vi "GxSingleCam.vi"() -> ()   [LabVIEW 2013]
uses:
  C:/Program Files/Daheng Imaging/GalaxySDK/Samples/LabVIEW SDK/x64/GxLVLib/dll/GxIAPINET.dll
  GxLVLib/dll/GxIAPINET.dll
  <vilib>/vision/Image Controls.llb/IMAQ Image.ctl
  GxLVLib/GxLVlib.lvlib
panel:
  out "IsExit":bool
  in  "Image Path":path
  in  "ImageSaving":bool
  in  "Image Src":T1
  out "Image":T1(plugin-control)
  out "Acquisition Callback":refnum<k27>
  out "IsColor":bool
  out "Acquisition Status":bool
  out "Open Status":bool
  in  "IGxFactory":refnum<k24>
  in  "Exit":bool
  in  "IGxStream":refnum<k24>
  in  "IGxDevice":refnum<k24>
  out "error out":errorcluster
  in  "TriggerSoftware":bool
  in  "BalanceWhiteAuto":string(combo)
  in  "Gain":dbl format="%#_6f"
  in  "ExposureTime":dbl
  in  "TriggerSource":string(combo)
  in  "TriggerMode":string(combo)
  in  "Acquisition Stop":bool
  in  "Acquisition Start":bool
  in  "Close Device":bool
  in  "Open Device":bool
  # "TriggerMode"
  # "TriggerSource"
  # "TriggerSoftware"
  # "ExposureTime(us)"
  # "Gain(dB)"
  # "BalanceWhiteAuto"
  # "ImageSaving"
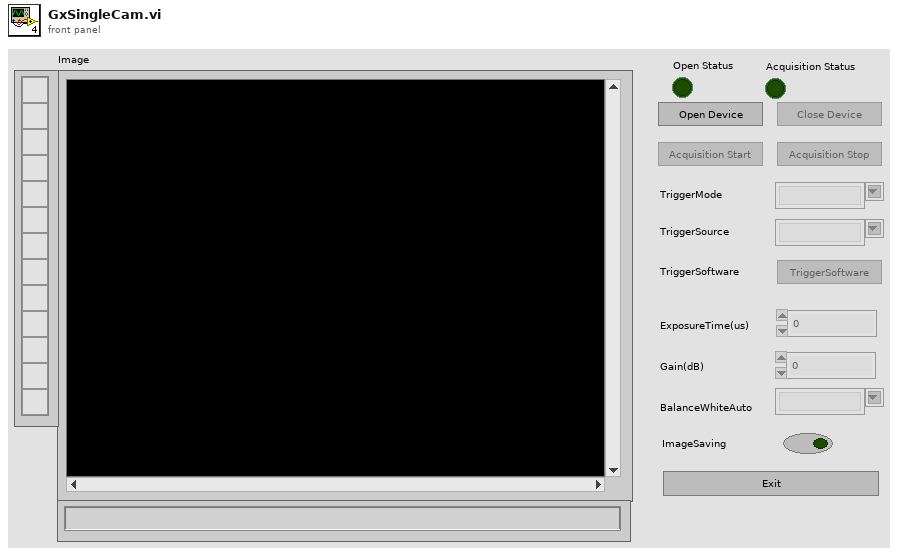
[diagram p1: front panel]
types:
  T1 = typedef "IMAQ Image.ctl" = refnum<image>
  T2 = typedef "Semaphore RefNum" = refnum<k1>
  T3 = enum8{"Enabled", "Disabled", "Disabled and Grayed Out"}
  T4 = typedef "Image Type" = u32
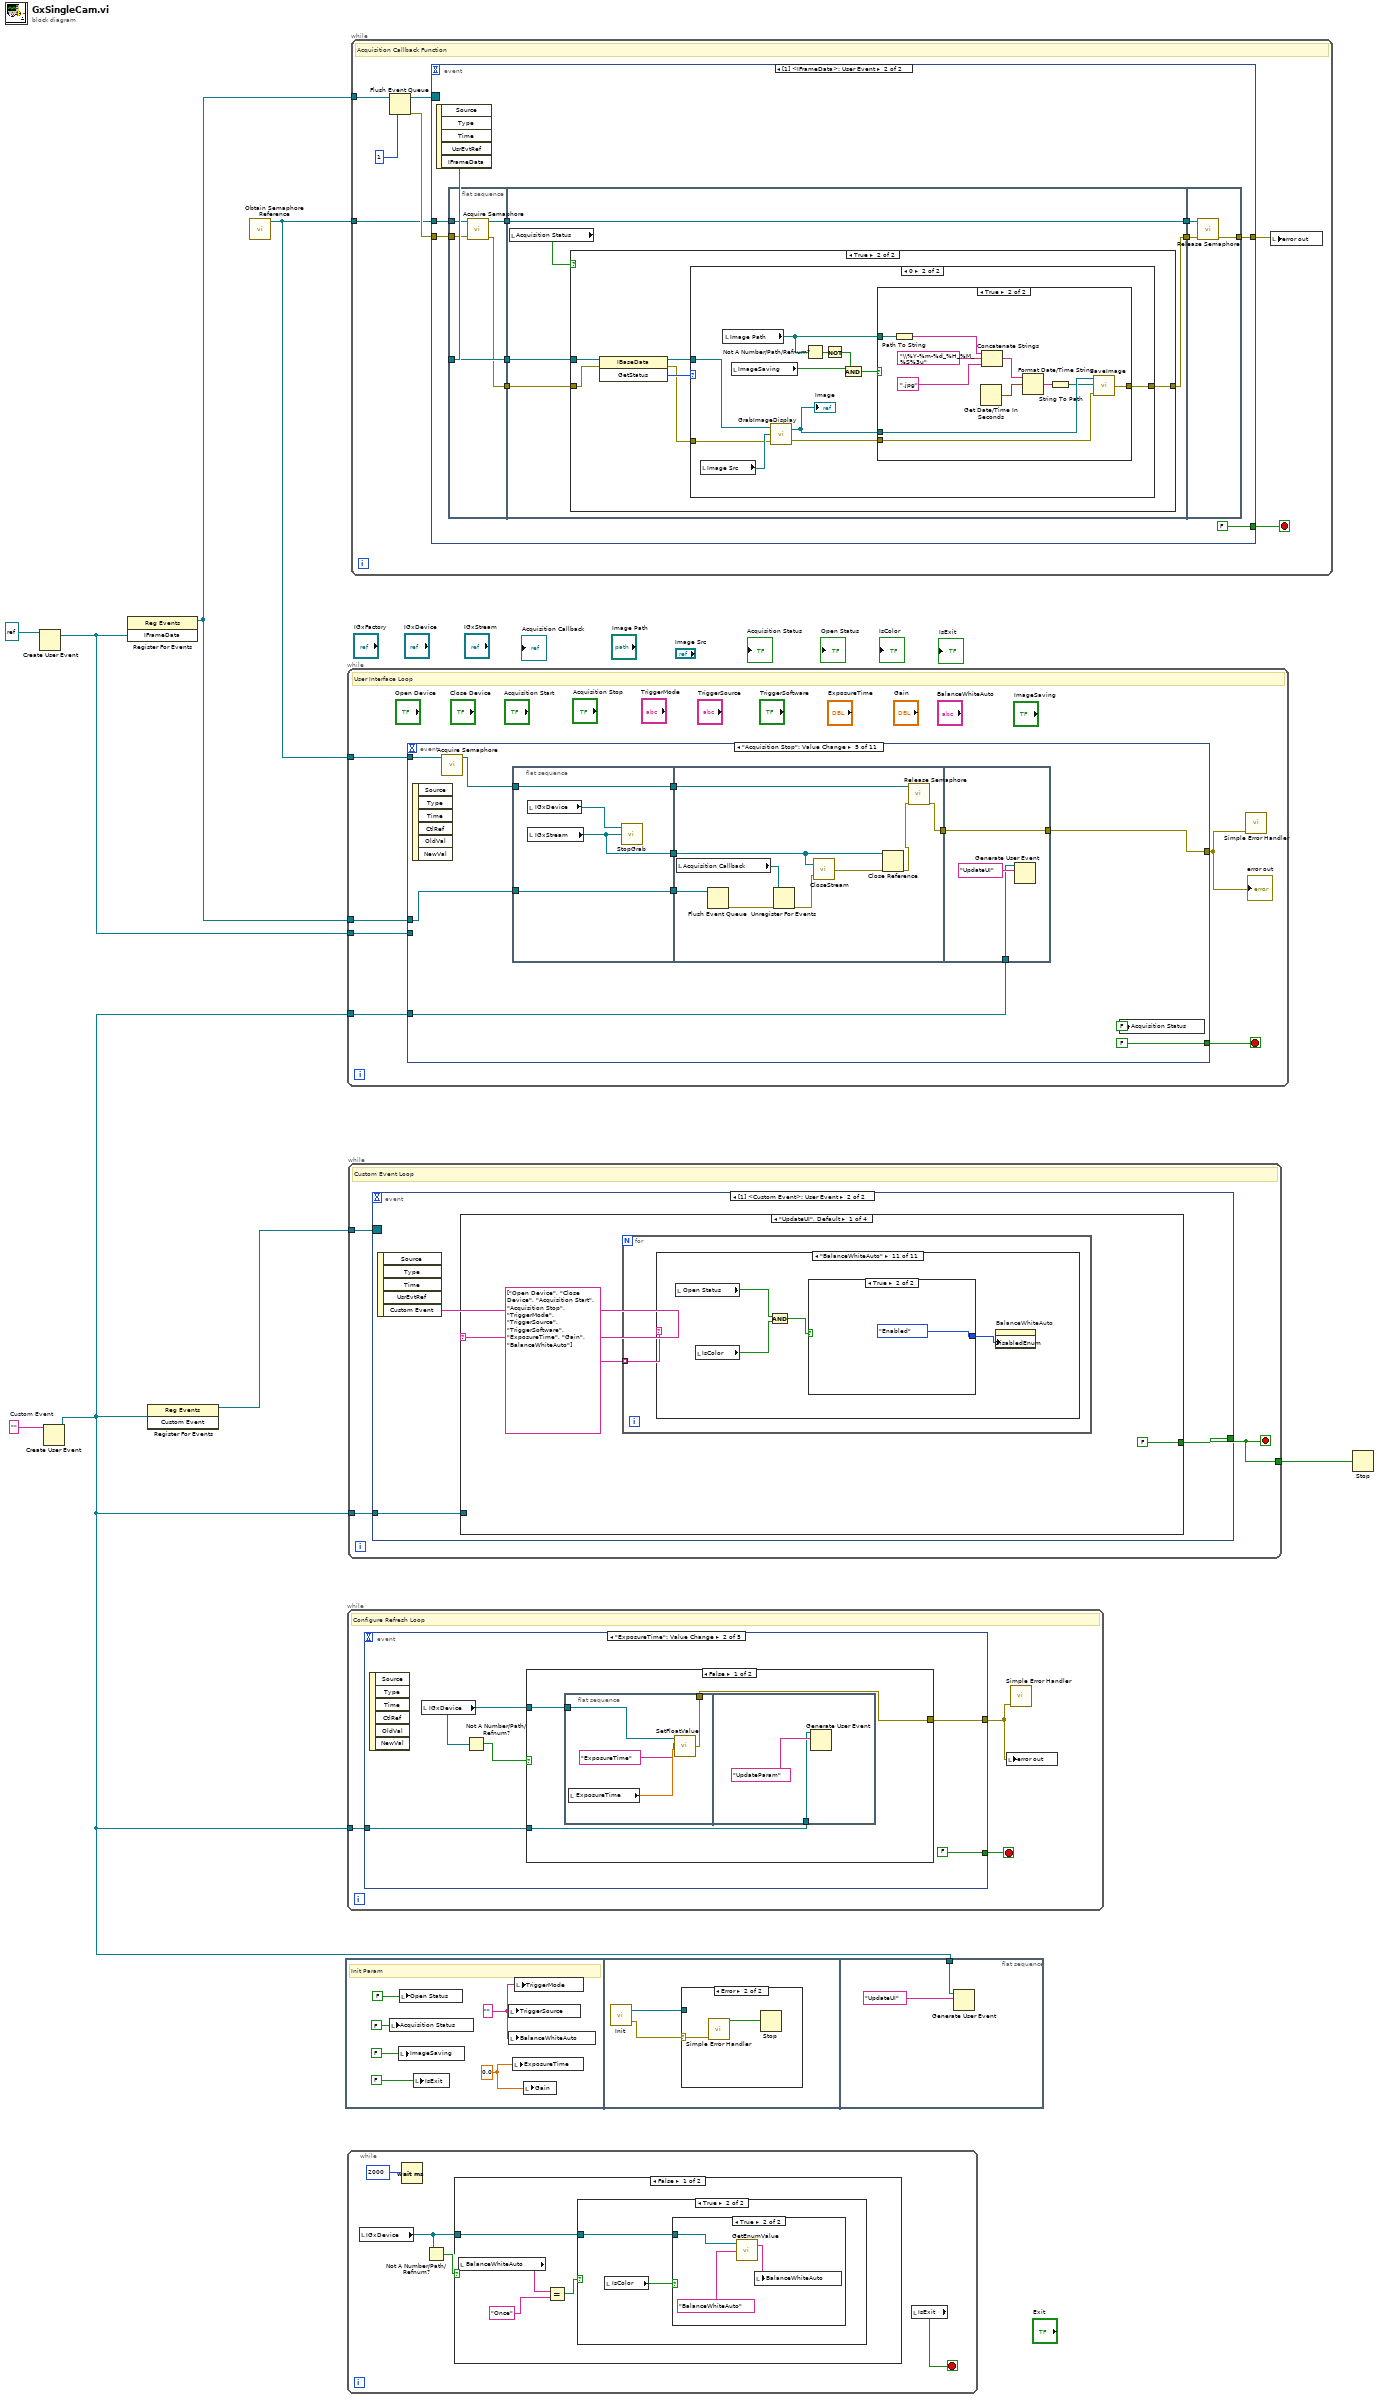
[diagram p0: block diagram]
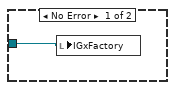
[diagram p5: hidden frame]
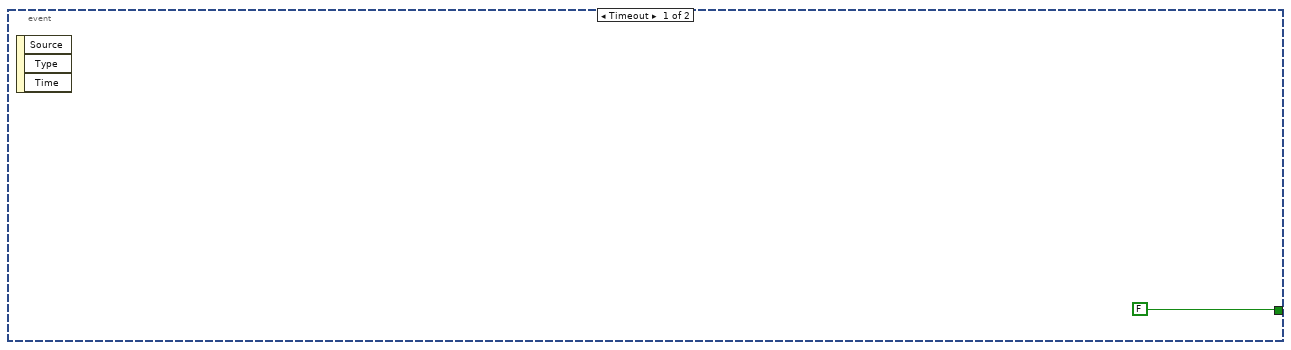
[diagram p6: hidden frame]
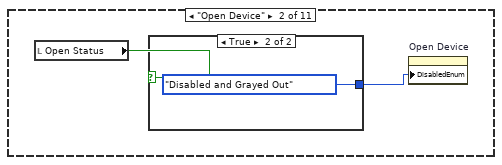
[diagram p8: hidden frame]
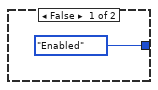
[diagram p9: hidden frame]
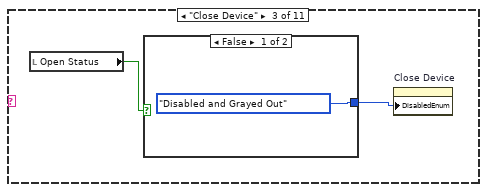
[diagram p10: hidden frame]
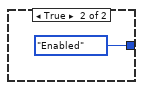
[diagram p11: hidden frame]
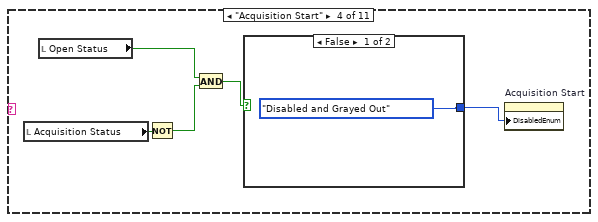
[diagram p12: hidden frame]
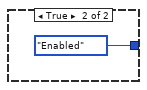
[diagram p13: hidden frame]
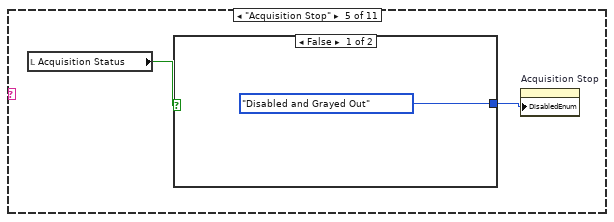
[diagram p14: hidden frame]
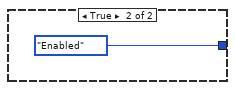
[diagram p15: hidden frame]
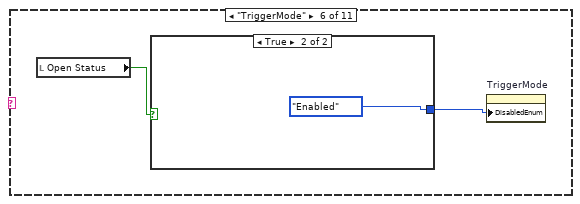
[diagram p16: hidden frame]
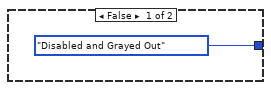
[diagram p17: hidden frame]
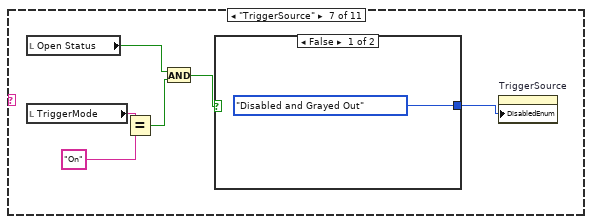
[diagram p18: hidden frame]
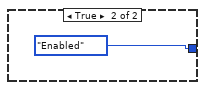
[diagram p19: hidden frame]
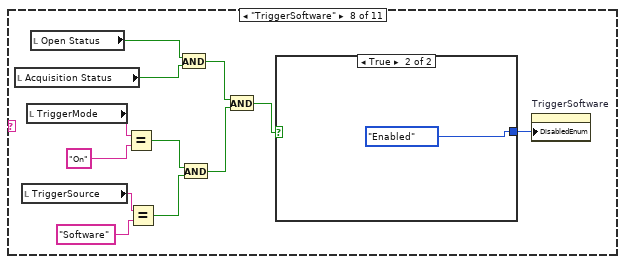
[diagram p20: hidden frame]
diagram:
  w6 = ""  # Custom Event
  n1 = Create User Event(user event datatype=refnum<k24> refnum ("IFrameData")) -> (user event=w8:refnum<user-event>)  [unwired: 1 in, 1 out]
  n2 = Create User Event(user event datatype=w6) -> (user event=w3:refnum<user-event>)  [unwired: 1 in, 1 out]
  n3 = register-events(w8) -> (reference out=w2:refnum<event-registration>)  [unwired: 2 in, 1 out]
  n4 = register-events(w3) -> (reference out=w5:refnum<event-registration>)  [unwired: 2 in, 1 out]
  n5 = call <vilib>:"Obtain Semaphore Reference.vi"() -> ("semaphore"=w1:T2)  [unwired: 5 in, 2 out]
  n6 = flat-sequence {
    tunnel: w3 -> [w20]
    frame #0 {
      w11 = 0.0
      w12 = ""
      # "Init Param"
      n7 = local write "Acquisition Status"(FALSE) -> ()
      n8 = local write "ImageSaving"(FALSE) -> ()
      n9 = local write "Open Status"(FALSE) -> ()
      n10 = local write "IsExit"(FALSE) -> ()
      n11 = local write "TriggerSource"(w12) -> ()
      n12 = local write "BalanceWhiteAuto"(w12) -> ()
      n13 = local write "ExposureTime"(w11) -> ()
      n14 = local write "TriggerMode"(w12) -> ()
      n15 = local write "Gain"(w11) -> ()
    }
    frame #1 {
      n16 = call "Init.vi"() -> ("IGxFactory"=w16:refnum<k24>, "error out"=w15:errorcluster)  [unwired: 1 in]
      n17 = case shown="Error" w15 {
        selector: w15 -> [_ w18]
        tunnel: w16 -> [w17 _]
        frame No Error {
          n18 = local write "IGxFactory"(w17) -> ()
        }
        frame Error {
          n19 = call <vilib>:"Simple Error Handler.vi"("error in (no error)"=w18) -> ("error?"=w19:bool)  [unwired: 4 in, 4 out]
          n20 = Stop(stop? (T)=w19) -> ()
        }
      }
    }
    frame #2 {
      n21 = Generate User Event(user event=w20, event data cluster="UpdateUI") -> ()  [unwired: 2 in, 2 out]
    }
  }
  n22 = while {
    tunnel: w3 -> [w22]
    stop <- w24 stop-if-true
    # "Configure Refresh Loop"
    n23 = event shown="[1] \"ExposureTime\": Value Change" {
      selector: _ -> [_ _ _ _ _]
      dyn-events: _ -> [_ _ _ _ _]
      timeout: _ -> [_ _ _ _ _]
      tunnel: [errorcluster {FALSE, 0, ""} w29 w44 w59 errorcluster {"status"=FALSE, "code"=0, "source"=""} ("错误常量")] -> w23
      tunnel: [FALSE FALSE FALSE FALSE TRUE] -> w24
      tunnel: w22 -> [_ w27 w42 w57 _]
      event Timeout {
        n24 = event-data() -> ()  [unwired: 1 in, 3 out]
      }
      event "ExposureTime": Value Change {
        n25 = event-data() -> ()  [unwired: 1 in, 6 out]
        n26 = local read "IGxDevice"() -> (w30:refnum<k24>)
        n27 = Not A Number/Path/Refnum?(number/path/refnum=w30) -> (NaN/Path/Refnum?=w31:bool)
        n28 = case shown="False" w31 {
          tunnel: w30 -> [w34 _]
          tunnel: [w33 errorcluster {TRUE, 5000, "GxSingleCam.vi"}] -> w29
          tunnel: w27 -> [w32 _]
          frame False {
            n29 = flat-sequence {
              tunnel: w34 -> [w36]
              tunnel: [w35] -> w33
              tunnel: w32 -> [w39]
              frame #0 {
                n30 = local read "ExposureTime"() -> (w38:dbl)
                n31 = call "SetFloatValue.vi"("Float Value"=w38, "Feature Name"="ExposureTime", "IGxDevice"=w36) -> ("error out"=w35:errorcluster)  [unwired: 1 in]
              }
              frame #1 {
                n32 = Generate User Event(user event=w39, event data cluster="UpdateParam") -> ()  [unwired: 2 in, 2 out]
              }
            }
          }
          frame True {
          }
        }
      }
      event "Gain": Value Change {
        n33 = event-data() -> ()  [unwired: 1 in, 6 out]
        n34 = local read "IGxDevice"() -> (w46:refnum<k24>)
        n35 = Not A Number/Path/Refnum?(number/path/refnum=w46) -> (NaN/Path/Refnum?=w45:bool)
        n36 = case shown="True" w45 {
          tunnel: w46 -> [w49 _]
          tunnel: [w48 errorcluster {TRUE, 0, "设备句柄无效"}] -> w44
          tunnel: w42 -> [w47 _]
          frame False {
            n37 = flat-sequence {
              tunnel: w49 -> [w51]
              tunnel: [w50] -> w48
              tunnel: w47 -> [w55]
              frame #0 {
                n38 = local read "Gain"() -> (w53:dbl)
                n39 = call "SetFloatValue.vi"("Float Value"=w53, "Feature Name"="Gain", "IGxDevice"=w51) -> ("error out"=w50:errorcluster)  [unwired: 1 in]
              }
              frame #1 {
                n40 = Generate User Event(user event=w55, event data cluster="UpdateParam") -> ()  [unwired: 2 in, 2 out]
              }
            }
          }
          frame True {
          }
        }
      }
      event "BalanceWhiteAuto": Value Change {
        n41 = event-data() -> ()  [unwired: 1 in, 6 out]
        n42 = local read "IGxDevice"() -> (w60:refnum<k24>)
        n43 = Not A Number/Path/Refnum?(number/path/refnum=w60) -> (NaN/Path/Refnum?=w61:bool)
        n44 = case shown="False" w61 {
          tunnel: w60 -> [w64 _]
          tunnel: [w63 errorcluster {TRUE, 0, "设备句柄无效"}] -> w59
          tunnel: w57 -> [w62 _]
          frame False {
            n45 = flat-sequence {
              tunnel: w64 -> [w66]
              tunnel: [w65] -> w63
              tunnel: w62 -> [w69]
              frame #0 {
                n46 = local read "BalanceWhiteAuto"() -> (w68:string)
                n47 = call "SetEnumValue.vi"("Enum Value"=w68, "Feature Name"="BalanceWhiteAuto", "IGxDevice"=w66) -> ("error out"=w65:errorcluster)  [unwired: 1 in]
              }
              frame #1 {
                n48 = Generate User Event(user event=w69, event data cluster="UpdateParam") -> ()  [unwired: 2 in, 2 out]
              }
            }
          }
          frame True {
          }
        }
      }
      event "Exit": Value Change {
        n49 = event-data() -> ()  [unwired: 1 in, 6 out]
      }
    }
    n50 = local write "error out"(w23) -> ()
    n51 = call <vilib>:"Simple Error Handler.vi"("error in (no error)"=w23) -> ()  [unwired: 4 in, 5 out]
  }
  n52 = while {
    stop <- w74 stop-if-true
    n53 = local read "IGxDevice"() -> (w76:refnum<k24>)
    n54 = Wait (ms)(milliseconds to wait=2000) -> ()  [unwired: 1 out]
    n55 = Not A Number/Path/Refnum?(number/path/refnum=w76) -> (NaN/Path/Refnum?=w75:bool)
    n56 = case shown="False" w75 {
      tunnel: w76 -> [w81 _]
      frame False {
        n57 = local read "BalanceWhiteAuto"() -> (w79:string)
        n58 = Equal?(x=w79, y="Once") -> (x = y?=w78:bool)
        n59 = case shown="True" w78 {
          tunnel: w81 -> [_ w82]
          frame False {
          }
          frame True {
            n60 = local read "IsColor"() -> (w83:bool)
            n61 = case shown="True" w83 {
              tunnel: w82 -> [_ w86]
              frame False {
              }
              frame True {
                n62 = call "GetEnumValue.vi"("Feature Name"="BalanceWhiteAuto", "IGxDevice"=w86) -> ("Enum Value"=w84:string)  [unwired: 1 in, 1 out]
                n63 = local write "BalanceWhiteAuto"(w84) -> ()
              }
            }
          }
        }
      }
      frame True {
      }
    }
    n64 = local read "IsExit"() -> (w74:bool)
  }
  n65 = while {
    tunnel: w8 -> [w92]
    tunnel: w3 -> [w91]
    tunnel: w2 -> [w88]
    tunnel: w1 -> [w87]
    stop <- w89 stop-if-true
    # "User Interface Loop"
    n66 = event shown="[4] \"Acquisition Stop\": Value Change" {
      selector: _ -> [_ _ _ _ _ _ _ _ _ _ _]
      dyn-events: _ -> [_ _ _ _ _ _ _ _ _ _ _]
      timeout: _ -> [_ _ _ _ _ _ _ _ _ _ _]
      tunnel: [errorcluster {FALSE, 0, ""} w97 _ w167 w197 w225 w233 w240 _ _ _] -> w90
      tunnel: [FALSE FALSE FALSE FALSE FALSE FALSE FALSE FALSE FALSE TRUE TRUE] -> w89
      tunnel: w92 -> [_ _ _ w168 _ _ _ _ _ _ _]
      tunnel: w91 -> [_ w95 w126 w165 w198 w227 w234 w242 _ w260 w302]
      tunnel: w88 -> [_ _ w125 _ w199 _ _ _ _ w261 w303]
      tunnel: w87 -> [_ _ w124 _ w206 _ _ _ _ w259 w301]
      event Timeout {
        n67 = event-data() -> ()  [unwired: 1 in, 3 out]
      }
      event "Open Device": Value Change {
        n68 = event-data() -> ()  [unwired: 1 in, 6 out]
        n69 = flat-sequence {
          tunnel: [w101] -> w96
          tunnel: [w123] -> w97
          tunnel: w96 -> [w123]
          tunnel: w95 -> [w120]
          frame #0 {
            n70 = local read "IGxFactory"() -> (w102:refnum<k24>)
            n71 = call "UpdateDeviceList.vi"("time out"=1000, "IGxFactory"=w102) -> ("error out"=w99:errorcluster, "DeviceSNList"=w100:string[])  [unwired: 1 in]
            n72 = Array Size(array=w100) -> (size(s)=w103:i32)
            n73 = case shown="Default" w103 {
              tunnel: w100 -> [w112 _]
              tunnel: w102 -> [w108 _]
              tunnel: [w107 w118] -> w101
              tunnel: w99 -> [w106 w119]
              frame Default {
                n74 = Index Array(array=w112, index=0) -> (element=w109:string)
                n75 = call "OpenDeviceBySN.vi"("error in (no error)"=w106, "SN"=w109, "IGxFactory"=w108) -> ("error out"=w105:errorcluster, "IGxDevice"=w110:refnum<k24>)
                n76 = case shown="No Error" w105 {
                  selector: w105 -> [w113 w116]
                  tunnel: w110 -> [w114 _]
                  tunnel: [w113 w116] -> w107
                  frame No Error {
                    n77 = local write "IGxDevice"(w114) -> ()
                    n78 = local write "Open Status"(TRUE) -> ()
                  }
                  frame Error {
                  }
                }
              }
              frame 0 {
                n79 = Merge Errors(w119, errorcluster {TRUE, 5001, "GxSingleCam.vi"}) -> (w118:errorcluster)
              }
            }
          }
          frame #1 {
            n80 = Generate User Event(user event=w120, event data cluster="UpdateParam") -> ()  [unwired: 2 in, 2 out]
            n81 = Generate User Event(user event=w120, event data cluster="PicShow") -> ()  [unwired: 2 in, 2 out]
          }
        }
      }
      event "Close Device": Value Change {
        n82 = event-data() -> ()  [unwired: 1 in, 6 out]
        n83 = flat-sequence {
          tunnel: w125 -> [w131]
          tunnel: w124 -> [w130]
          tunnel: w126 -> [w163]
          frame #0 {
            n84 = local read "IGxStream"() -> (w135:refnum<k24>)
            n85 = local read "IGxDevice"() -> (w134:refnum<k24>)
            n86 = Not A Number/Path/Refnum?(number/path/refnum=w135) -> (NaN/Path/Refnum?=w136:bool)
            n87 = case shown="False" w136 {
              tunnel: w135 -> [w149 _]
              tunnel: w134 -> [w147 w162]
              tunnel: w131 -> [w144 _]
              tunnel: [w146 w162] -> w132
              tunnel: w130 -> [w142 _]
              frame False {
                n88 = call <vilib>:"Acquire Semaphore.vi"("semaphore"=w142) -> ("semaphore out"=w141:T2)  [unwired: 4 in, 2 out]
                n89 = flat-sequence {
                  tunnel: w149 -> [w152]
                  tunnel: [w153] -> w148
                  tunnel: w147 -> [w153]
                  tunnel: [w151] -> w145
                  tunnel: w144 -> [w151]
                  tunnel: [w152] -> w143
                  tunnel: w141 -> [w150]
                  tunnel: [w150] -> w140
                  tunnel: w148 -> [w161]
                  tunnel: [w161] -> w146
                  tunnel: w145 -> [w160]
                  tunnel: w143 -> [w156]
                  tunnel: [w154] -> w139
                  tunnel: w140 -> [w154]
                  frame #0 {
                    n90 = call "StopGrab.vi"("IGxStream"=w152, "IGxDevice"=w153) -> ()  [unwired: 1 in, 1 out]
                  }
                  frame #1 {
                    n91 = local read "Acquisition Callback"() -> (w158:refnum<k27>)
                    n92 = Flush Event Queue(0:w160) -> (11:w159:errorcluster)  [unwired: 5 in, 2 out]
                    n93 = Unregister For Events(event registration refnum=w158, error in=w159) -> (error out=w155:errorcluster)
                    n94 = call "CloseStream.vi"("error in (no error)"=w155, "IGxStream"=w156) -> ("error out"=w157:errorcluster)
                    n95 = Close Reference(reference=w156, error in (no error)=w157) -> ()  [unwired: 1 out]
                  }
                }
                n96 = call <vilib>:"Release Semaphore.vi"("semaphore"=w139) -> ()  [unwired: 5 in, 2 out]
              }
              frame True {
              }
            }
            n97 = local read "Image Src"() -> (w137:T1)
            n98 = call "CloseDevice.vi"("IGxDevice"=w132) -> ("error out"=w138:errorcluster)  [unwired: 1 in]
            n99 = Close Reference(reference=w132, error in (no error)=w138) -> (error out=w133:errorcluster)
            n100 = call "Imaq Dispose"("Image"=w137, "error in (no error)"=w133) -> ()  [unwired: 1 in, 4 out]
          }
          frame #1 {
            n101 = Generate User Event(user event=w163, event data cluster="UpdateUI") -> ()  [unwired: 2 in, 2 out]
          }
        }
        n102 = local write "Acquisition Status"(FALSE) -> ()
        n103 = local write "Open Status"(FALSE) -> ()
      }
      event "Acquisition Start": Value Change {
        n104 = event-data() -> ()  [unwired: 1 in, 6 out]
        n105 = flat-sequence {
          tunnel: w168 -> [w177]
          tunnel: [w171] -> w166
          tunnel: [w196] -> w167
          tunnel: w166 -> [w196]
          tunnel: w165 -> [w194]
          frame #0 {
            n106 = local read "IGxDevice"() -> (w179:refnum<k24>)
            n107 = vi-ref "ImageGrabEvent.vi"() -> (w172:refnum<vi>)
            n108 = call "OpenStream.vi"("StreamID"=0, "IGxDevice"=w179) -> ("error out"=w176:errorcluster, "IGxStream"=w174:refnum<k24>)  [unwired: 1 in]
            n109 = node(w176, w174, w172, w177) -> (w173:refnum<k27>, w175:errorcluster)  [unwired: 1 in]
            n110 = local write "Acquisition Callback"(w173) -> ()
            n111 = local write "IGxStream"(w174) -> ()
            n112 = call "StartGrab.vi"("error in (no error)"=w175, "IGxStream"=w174, "IGxDevice"=w179) -> ("error out"=w170:errorcluster)
            n113 = case shown="Error" w170 {
              selector: w170 -> [w180 w183]
              tunnel: w174 -> [_ w187]
              tunnel: w173 -> [_ w188]
              tunnel: [w180 w184] -> w171
              frame No Error {
                n114 = local write "Acquisition Status"(TRUE) -> ()
              }
              frame Error {
                n115 = Not A Number/Path/Refnum?(number/path/refnum=w188) -> (NaN/Path/Refnum?=w189:bool)
                n116 = call "CloseStream.vi"("IGxStream"=w187) -> ("error out"=w186:errorcluster)  [unwired: 1 in]
                n117 = Close Reference(reference=w187, error in (no error)=w186) -> (error out=w185:errorcluster)
                n118 = case shown="False" w189 {
                  tunnel: w188 -> [w192 _]
                  tunnel: [w191 w193] -> w182
                  tunnel: w185 -> [w190 w193]
                  frame False {
                    n119 = Unregister For Events(event registration refnum=w192, error in=w190) -> (error out=w191:errorcluster)
                  }
                  frame True {
                  }
                }
                n120 = Merge Errors(w183, w182) -> (w184:errorcluster)
              }
            }
          }
          frame #1 {
            n121 = Generate User Event(user event=w194, event data cluster="UpdateUI") -> ()  [unwired: 2 in, 2 out]
          }
        }
      }
      event "Acquisition Stop": Value Change {
        n122 = event-data() -> ()  [unwired: 1 in, 6 out]
        n123 = call <vilib>:"Acquire Semaphore.vi"("semaphore"=w206) -> ("semaphore out"=w201:T2)  [unwired: 4 in, 2 out]
        n124 = flat-sequence {
          tunnel: [w208] -> w204
          tunnel: [w210] -> w203
          tunnel: w201 -> [w209]
          tunnel: [w209] -> w200
          tunnel: w199 -> [w208]
          tunnel: [w213] -> w202
          tunnel: w204 -> [w220]
          tunnel: w203 -> [w216]
          tunnel: w200 -> [w212]
          tunnel: [w223] -> w197
          tunnel: w202 -> [w223]
          tunnel: w198 -> [w221]
          frame #0 {
            n125 = local read "IGxDevice"() -> (w211:refnum<k24>)
            n126 = local read "IGxStream"() -> (w210:refnum<k24>)
            n127 = call "StopGrab.vi"("IGxStream"=w210, "IGxDevice"=w211) -> ()  [unwired: 1 in, 1 out]
          }
          frame #1 {
            n128 = local read "Acquisition Callback"() -> (w219:refnum<k27>)
            n129 = Flush Event Queue(0:w220) -> (11:w218:errorcluster)  [unwired: 5 in, 2 out]
            n130 = Unregister For Events(event registration refnum=w219, error in=w218) -> (error out=w215:errorcluster)
            n131 = call "CloseStream.vi"("error in (no error)"=w215, "IGxStream"=w216) -> ("error out"=w217:errorcluster)
            n132 = Close Reference(reference=w216, error in (no error)=w217) -> (error out=w214:errorcluster)
            n133 = call <vilib>:"Release Semaphore.vi"("error in (no error)"=w214, "semaphore"=w212) -> ("error out"=w213:errorcluster)  [unwired: 4 in, 1 out]
          }
          frame #2 {
            n134 = Generate User Event(user event=w221, event data cluster="UpdateUI") -> ()  [unwired: 2 in, 2 out]
          }
        }
        n135 = local write "Acquisition Status"(FALSE) -> ()
      }
      event "TriggerMode": Value Change {
        n136 = event-data() -> ()  [unwired: 1 in, 6 out]
        n137 = local read "TriggerMode"() -> (w230:string)
        n138 = local read "IGxDevice"() -> (w231:refnum<k24>)
        n139 = call "SetEnumValue.vi"("Enum Value"=w230, "Feature Name"="TriggerMode", "IGxDevice"=w231) -> ("error out"=w226:errorcluster)  [unwired: 1 in]
        n140 = Generate User Event(user event=w227, event data cluster="UpdateParam", error in=w226) -> (error out=w225:errorcluster)  [unwired: 1 in, 1 out]
      }
      event "TriggerSource": Value Change {
        n141 = event-data() -> ()  [unwired: 1 in, 6 out]
        n142 = local read "TriggerSource"() -> (w237:string)
        n143 = local read "IGxDevice"() -> (w239:refnum<k24>)
        n144 = call "SetEnumValue.vi"("Enum Value"=w237, "Feature Name"="TriggerSource", "IGxDevice"=w239) -> ("error out"=w235:errorcluster)  [unwired: 1 in]
        n145 = Generate User Event(user event=w234, event data cluster="UpdateUI", error in=w235) -> (error out=w233:errorcluster)  [unwired: 1 in, 1 out]
      }
      event "TriggerSoftware": Value Change {
        n146 = event-data() -> ()  [unwired: 1 in, 6 out]
        n147 = local read "IGxDevice"() -> (w246:refnum<k24>)
        n148 = call "SetCommandValue.vi"("Feature Name"="TriggerSoftware", "IGxDevice"=w246) -> ("error out"=w243:errorcluster)  [unwired: 1 in]
        n149 = Generate User Event(user event=w242, event data cluster="UpdateUI", error in=w243) -> (error out=w240:errorcluster)  [unwired: 1 in, 1 out]
      }
      event "ImageSaving": Value Change {
        n150 = event-data() -> ()  [unwired: 1 in, 6 out]
        n151 = local read "ImageSaving"() -> (w248:bool)
        n152 = case shown="True" w248 {
          frame False {
          }
          frame True {
            n153 = call <vilib>:"Application Directory.vi"() -> ("Application Directory"=w255:path)
            n154 = Path To String(path=w255) -> (string=w254:string)
            n155 = Concatenate Strings(w254, "\\Image") -> (w252:string)
            n156 = String To Path(string=w252) -> (path=w250:path)
            n157 = call <vilib>:"Check if File or Folder Exists.vi"("path"=w250) -> ("file or folder exists?"=w251:bool)  [unwired: 8 in, 2 out]
            n158 = case shown="False" w251 {
              tunnel: w250 -> [w257 w258]
              tunnel: [w256 w258] -> w249
              frame False {
                n159 = Create Folder(path (use dialog)=w257) -> (created path=w256:path)  [unwired: 2 in, 2 out]
              }
              frame True {
              }
            }
            n160 = local write "Image Path"(w249) -> ()
          }
        }
      }
      event "Exit": Value Change {
        n161 = event-data() -> ()  [unwired: 1 in, 6 out]
        n162 = flat-sequence {
          tunnel: w261 -> [w266]
          tunnel: w259 -> [w263]
          tunnel: w260 -> [w299]
          frame #0 {
            n163 = local read "Acquisition Status"() -> (w267:bool)
            n164 = local read "IGxDevice"() -> (w265:refnum<k24>)
            n165 = local read "IGxStream"() -> (w268:refnum<k24>)
            n166 = case shown="True" w267 {
              tunnel: w268 -> [_ w284]
              tunnel: w266 -> [_ w280]
              tunnel: w265 -> [w273 w283]
              tunnel: [w273 w279] -> w264
              tunnel: w263 -> [_ w277]
              frame False {
              }
              frame True {
                n167 = call <vilib>:"Acquire Semaphore.vi"("semaphore"=w277) -> ("semaphore out"=w276:T2)  [unwired: 4 in, 2 out]
                n168 = flat-sequence {
                  tunnel: w284 -> [w286]
                  tunnel: w283 -> [w288]
                  tunnel: [w288] -> w282
                  tunnel: [w287] -> w281
                  tunnel: w280 -> [w287]
                  tunnel: [w286] -> w278
                  tunnel: w276 -> [w285]
                  tunnel: [w285] -> w275
                  tunnel: [w297] -> w279
                  tunnel: w282 -> [w297]
                  tunnel: w281 -> [w296]
                  tunnel: w278 -> [w292]
                  tunnel: [w289] -> w274
                  tunnel: w275 -> [w289]
                  frame #0 {
                    n169 = call "StopGrab.vi"("IGxStream"=w286, "IGxDevice"=w288) -> ()  [unwired: 1 in, 1 out]
                  }
                  frame #1 {
                    n170 = local read "Acquisition Callback"() -> (w294:refnum<k27>)
                    n171 = Flush Event Queue(0:w296) -> (11:w295:errorcluster)  [unwired: 5 in, 2 out]
                    n172 = local write "Acquisition Status"(FALSE) -> ()
                    n173 = Unregister For Events(event registration refnum=w294, error in=w295) -> (error out=w291:errorcluster)
                    n174 = call "CloseStream.vi"("error in (no error)"=w291) -> ("error out"=w293:errorcluster)  [unwired: 1 in]
                    n175 = Close Reference(reference=w292, error in (no error)=w293) -> ()  [unwired: 1 out]
                  }
                }
                n176 = call <vilib>:"Release Semaphore.vi"("semaphore"=w274) -> ()  [unwired: 5 in, 2 out]
              }
            }
            n177 = local read "Open Status"() -> (w269:bool)
            n178 = case shown="True" w269 {
              tunnel: w264 -> [_ w270]
              frame False {
              }
              frame True {
                n179 = call "CloseDevice.vi"("IGxDevice"=w270) -> ("error out"=w272:errorcluster)  [unwired: 1 in]
                n180 = local write "Open Status"(FALSE) -> ()
                n181 = Close Reference(reference=w270, error in (no error)=w272) -> ()  [unwired: 1 out]
              }
            }
          }
          frame #1 {
            n182 = local write "IsExit"(TRUE) -> ()
            n183 = Generate User Event(user event=w299, event data cluster="Quit") -> ()  [unwired: 2 in, 2 out]
          }
        }
      }
      event Panel Close? {
        n184 = event-data() -> ()  [unwired: 1 in, 4 out]
        n185 = flat-sequence {
          tunnel: w303 -> [w306]
          tunnel: w301 -> [w305]
          tunnel: w302 -> [w340]
          frame #0 {
            n186 = local read "Acquisition Status"() -> (w309:bool)
            n187 = local read "IGxDevice"() -> (w308:refnum<k24>)
            n188 = local read "IGxStream"() -> (w310:refnum<k24>)
            n189 = case shown="True" w309 {
              tunnel: w310 -> [_ w326]
              tunnel: w306 -> [_ w322]
              tunnel: w308 -> [w315 w325]
              tunnel: [w315 w321] -> w307
              tunnel: w305 -> [_ w319]
              frame False {
              }
              frame True {
                n190 = call <vilib>:"Acquire Semaphore.vi"("semaphore"=w319) -> ("semaphore out"=w318:T2)  [unwired: 4 in, 2 out]
                n191 = flat-sequence {
                  tunnel: w326 -> [w328]
                  tunnel: w325 -> [w330]
                  tunnel: [w330] -> w324
                  tunnel: [w329] -> w323
                  tunnel: w322 -> [w329]
                  tunnel: [w328] -> w320
                  tunnel: w318 -> [w327]
                  tunnel: [w327] -> w317
                  tunnel: [w339] -> w321
                  tunnel: w324 -> [w339]
                  tunnel: w323 -> [w338]
                  tunnel: w320 -> [w334]
                  tunnel: [w331] -> w316
                  tunnel: w317 -> [w331]
                  frame #0 {
                    n192 = call "StopGrab.vi"("IGxStream"=w328, "IGxDevice"=w330) -> ()  [unwired: 1 in, 1 out]
                  }
                  frame #1 {
                    n193 = local read "Acquisition Callback"() -> (w336:refnum<k27>)
                    n194 = Flush Event Queue(0:w338) -> (11:w337:errorcluster)  [unwired: 5 in, 2 out]
                    n195 = local write "Acquisition Status"(FALSE) -> ()
                    n196 = Unregister For Events(event registration refnum=w336, error in=w337) -> (error out=w333:errorcluster)
                    n197 = call "CloseStream.vi"("error in (no error)"=w333) -> ("error out"=w335:errorcluster)  [unwired: 1 in]
                    n198 = Close Reference(reference=w334, error in (no error)=w335) -> ()  [unwired: 1 out]
                  }
                }
                n199 = call <vilib>:"Release Semaphore.vi"("semaphore"=w316) -> ()  [unwired: 5 in, 2 out]
              }
            }
            n200 = local read "Open Status"() -> (w311:bool)
            n201 = case shown="True" w311 {
              tunnel: w307 -> [_ w312]
              frame False {
              }
              frame True {
                n202 = call "CloseDevice.vi"("IGxDevice"=w312) -> ("error out"=w314:errorcluster)  [unwired: 1 in]
                n203 = local write "Open Status"(FALSE) -> ()
                n204 = Close Reference(reference=w312, error in (no error)=w314) -> ()  [unwired: 1 out]
              }
            }
          }
          frame #1 {
            n205 = local write "IsExit"(TRUE) -> ()
            n206 = Generate User Event(user event=w340, event data cluster="Quit") -> ()  [unwired: 2 in, 2 out]
          }
        }
        n207 = event-data() -> ()  [unwired: 2 in, 1 out]
      }
    }
    "error out" <- w90
    n208 = call <vilib>:"Simple Error Handler.vi"("error in (no error)"=w90) -> ()  [unwired: 4 in, 5 out]
  }
  n209 = while {
    tunnel: w5 -> [w345]
    tunnel: w3 -> [w344]
    tunnel: [w343] -> w4
    stop <- w343 stop-if-true
    # "Custom Event Loop"
    n210 = event shown="[1] <Custom Event>: User Event" {
      selector: w345 -> [_ _]
      dyn-events: _ -> [_ _]
      timeout: _ -> [_ _]
      tunnel: [FALSE w347] -> w343
      tunnel: w344 -> [_ w348]
      event Timeout {
        n211 = event-data() -> ()  [unwired: 1 in, 3 out]
      }
      event User Event {
        n212 = event-data() -> ("Custom Event"=w349:string)  [unwired: 1 in, 4 out]
        n213 = case shown="\"UpdateUI\", Default" w349 {
          tunnel: w348 -> [_ _ w480 _]
          tunnel: [FALSE TRUE FALSE FALSE] -> w347
          frame "UpdateUI", Default {
            n214 = for {
              tunnel: string[] ["Open Device", "Close Device", "Acquisition Start", "Acquisition Stop", "TriggerMode", "TriggerSource", "TriggerSoftware", "ExposureTime", "Gain", "BalanceWhiteAuto"] -> [w352] mode=indexing
              n215 = case shown="\"BalanceWhiteAuto\"" w352 {
                frame Default {
                }
                frame "Open Device" {
                  n216 = local read "Open Status"() -> (w354:bool)
                  n217 = case shown="True" w354 {
                    tunnel: [T3."Enabled" ("禁用") T3."Disabled and Grayed Out" ("禁用")] -> w353
                    frame False {
                    }
                    frame True {
                    }
                  }
                  n218 = property on="Open Device" class="Bool"("DisabledEnum"=w353) -> ()  [unwired: 2 in, 2 out]
                }
                frame "Close Device" {
                  n219 = local read "Open Status"() -> (w358:bool)
                  n220 = case shown="False" w358 {
                    tunnel: [T3."Disabled and Grayed Out" ("禁用") T3."Enabled" ("禁用")] -> w357
                    frame False {
                    }
                    frame True {
                    }
                  }
                  n221 = property on="Close Device" class="Bool"("DisabledEnum"=w357) -> ()  [unwired: 2 in, 2 out]
                }
                frame "Acquisition Start" {
                  n222 = local read "Acquisition Status"() -> (w365:bool)
                  n223 = local read "Open Status"() -> (w364:bool)
                  n224 = Not(x=w365) -> (.not. x?=w363:bool)
                  n225 = And(x=w364, y=w363) -> (x .and. y?=w362:bool)
                  n226 = case shown="False" w362 {
                    tunnel: [T3."Disabled and Grayed Out" ("禁用") T3."Enabled" ("禁用")] -> w361
                    frame False {
                    }
                    frame True {
                    }
                  }
                  n227 = property on="Acquisition Start" class="Bool"("DisabledEnum"=w361) -> ()  [unwired: 2 in, 2 out]
                }
                frame "Acquisition Stop" {
                  n228 = local read "Acquisition Status"() -> (w369:bool)
                  n229 = case shown="False" w369 {
                    tunnel: [T3."Disabled and Grayed Out" ("禁用") T3."Enabled" ("禁用")] -> w368
                    frame False {
                    }
                    frame True {
                    }
                  }
                  n230 = property on="Acquisition Stop" class="Bool"("DisabledEnum"=w368) -> ()  [unwired: 2 in, 2 out]
                }
                frame "TriggerMode" {
                  n231 = local read "Open Status"() -> (w373:bool)
                  n232 = case shown="True" w373 {
                    tunnel: [T3."Disabled and Grayed Out" ("禁用") T3."Enabled" ("禁用")] -> w372
                    frame False {
                    }
                    frame True {
                    }
                  }
                  n233 = property on="TriggerMode" class="CmbBox"("DisabledEnum"=w372) -> ()  [unwired: 2 in, 2 out]
                }
                frame "TriggerSource" {
                  n234 = local read "Open Status"() -> (w379:bool)
                  n235 = local read "TriggerMode"() -> (w381:string)
                  n236 = Equal?(x=w381, y="On") -> (x = y?=w378:bool)
                  n237 = And(x=w379, y=w378) -> (x .and. y?=w377:bool)
                  n238 = case shown="False" w377 {
                    tunnel: [T3."Disabled and Grayed Out" ("禁用") T3."Enabled" ("禁用")] -> w376
                    frame False {
                    }
                    frame True {
                    }
                  }
                  n239 = property on="TriggerSource" class="CmbBox"("DisabledEnum"=w376) -> ()  [unwired: 2 in, 2 out]
                }
                frame "TriggerSoftware" {
                  n240 = local read "Acquisition Status"() -> (w385:bool)
                  n241 = local read "TriggerSource"() -> (w393:string)
                  n242 = local read "TriggerMode"() -> (w395:string)
                  n243 = local read "Open Status"() -> (w386:bool)
                  n244 = Equal?(x=w395, y="On") -> (x = y?=w391:bool)
                  n245 = Equal?(x=w393, y="Software") -> (x = y?=w390:bool)
                  n246 = And(x=w386, y=w385) -> (x .and. y?=w384:bool)
                  n247 = And(x=w391, y=w390) -> (x .and. y?=w389:bool)
                  n248 = And(x=w384, y=w389) -> (x .and. y?=w388:bool)
                  n249 = case shown="True" w388 {
                    tunnel: [T3."Disabled and Grayed Out" ("禁用") T3."Enabled" ("禁用")] -> w387
                    frame False {
                    }
                    frame True {
                    }
                  }
                  n250 = property on="TriggerSoftware" class="Bool"("DisabledEnum"=w387) -> ()  [unwired: 2 in, 2 out]
                }
                frame "ExposureTime" {
                  n251 = local read "Open Status"() -> (w399:bool)
                  n252 = case shown="False" w399 {
                    tunnel: [T3."Disabled and Grayed Out" ("禁用") T3."Enabled" ("禁用")] -> w398
                    frame False {
                    }
                    frame True {
                    }
                  }
                  n253 = property on="ExposureTime" class="DigNum (strict)"("DisabledEnum"=w398) -> ()  [unwired: 2 in, 2 out]
                }
                frame "Gain" {
                  n254 = local read "Open Status"() -> (w403:bool)
                  n255 = case shown="True" w403 {
                    tunnel: [T3."Disabled and Grayed Out" ("禁用") T3."Enabled" ("禁用")] -> w402
                    frame False {
                    }
                    frame True {
                    }
                  }
                  n256 = property on="Gain" class="DigNum (strict)"("DisabledEnum"=w402) -> ()  [unwired: 2 in, 2 out]
                }
                frame "BalanceWhiteAuto" {
                  n257 = local read "Open Status"() -> (w408:bool)
                  n258 = local read "IsColor"() -> (w409:bool)
                  n259 = And(x=w408, y=w409) -> (x .and. y?=w407:bool)
                  n260 = case shown="True" w407 {
                    tunnel: [T3."Disabled and Grayed Out" ("禁用") T3."Enabled" ("禁用")] -> w406
                    frame False {
                    }
                    frame True {
                    }
                  }
                  n261 = property on="BalanceWhiteAuto" class="CmbBox"("DisabledEnum"=w406) -> ()  [unwired: 2 in, 2 out]
                }
              }
            }
          }
          frame "Quit" {
            n262 = for {
              tunnel: string[] ["打开设备", "关闭设备", "开始采集", "停止采集", "触发模式", "触发源", "软触发", "曝光时间", "增益", "自动白平衡"] -> [w416] mode=indexing
              n263 = case shown="\"停止采集\"" w416 {
                frame Default {
                }
                frame "打开设备" {
                  n264 = local read "Open Status"() -> (w418:bool)
                  n265 = case shown="True" w418 {
                    tunnel: [T3."Enabled" ("禁用") T3."Disabled and Grayed Out" ("禁用")] -> w417
                    frame False {
                    }
                    frame True {
                    }
                  }
                  n266 = property on="Open Device" class="Bool"("DisabledEnum"=w417) -> ()  [unwired: 2 in, 2 out]
                }
                frame "关闭设备" {
                  n267 = local read "Open Status"() -> (w422:bool)
                  n268 = case shown="False" w422 {
                    tunnel: [T3."Disabled and Grayed Out" ("禁用") T3."Enabled" ("禁用")] -> w421
                    frame False {
                    }
                    frame True {
                    }
                  }
                  n269 = property on="Close Device" class="Bool"("DisabledEnum"=w421) -> ()  [unwired: 2 in, 2 out]
                }
                frame "开始采集" {
                  n270 = local read "Acquisition Status"() -> (w429:bool)
                  n271 = local read "Open Status"() -> (w428:bool)
                  n272 = Not(x=w429) -> (.not. x?=w427:bool)
                  n273 = And(x=w428, y=w427) -> (x .and. y?=w426:bool)
                  n274 = case shown="False" w426 {
                    tunnel: [T3."Disabled and Grayed Out" ("禁用") T3."Enabled" ("禁用")] -> w425
                    frame False {
                    }
                    frame True {
                    }
                  }
                  n275 = property on="Acquisition Start" class="Bool"("DisabledEnum"=w425) -> ()  [unwired: 2 in, 2 out]
                }
                frame "停止采集" {
                  n276 = local read "Acquisition Status"() -> (w433:bool)
                  n277 = case shown="False" w433 {
                    tunnel: [T3."Disabled and Grayed Out" ("禁用") T3."Enabled" ("禁用")] -> w432
                    frame False {
                    }
                    frame True {
                    }
                  }
                  n278 = property on="Acquisition Stop" class="Bool"("DisabledEnum"=w432) -> ()  [unwired: 2 in, 2 out]
                }
                frame "触发模式" {
                  n279 = local read "Open Status"() -> (w437:bool)
                  n280 = case shown="True" w437 {
                    tunnel: [T3."Disabled and Grayed Out" ("禁用") T3."Enabled" ("禁用")] -> w436
                    frame False {
                    }
                    frame True {
                    }
                  }
                  n281 = property on="TriggerMode" class="CmbBox"("DisabledEnum"=w436) -> ()  [unwired: 2 in, 2 out]
                }
                frame "触发源" {
                  n282 = local read "Open Status"() -> (w443:bool)
                  n283 = local read "TriggerMode"() -> (w445:string)
                  n284 = Equal?(x=w445, y="On") -> (x = y?=w442:bool)
                  n285 = And(x=w443, y=w442) -> (x .and. y?=w441:bool)
                  n286 = case shown="False" w441 {
                    tunnel: [T3."Disabled and Grayed Out" ("禁用") T3."Enabled" ("禁用")] -> w440
                    frame False {
                    }
                    frame True {
                    }
                  }
                  n287 = property on="TriggerSource" class="CmbBox"("DisabledEnum"=w440) -> ()  [unwired: 2 in, 2 out]
                }
                frame "软触发" {
                  n288 = local read "Acquisition Status"() -> (w449:bool)
                  n289 = local read "TriggerSource"() -> (w457:string)
                  n290 = local read "TriggerMode"() -> (w459:string)
                  n291 = local read "Open Status"() -> (w450:bool)
                  n292 = Equal?(x=w459, y="On") -> (x = y?=w455:bool)
                  n293 = Equal?(x=w457, y="Software") -> (x = y?=w454:bool)
                  n294 = And(x=w450, y=w449) -> (x .and. y?=w448:bool)
                  n295 = And(x=w455, y=w454) -> (x .and. y?=w453:bool)
                  n296 = And(x=w448, y=w453) -> (x .and. y?=w452:bool)
                  n297 = case shown="True" w452 {
                    tunnel: [T3."Disabled and Grayed Out" ("禁用") T3."Enabled" ("禁用")] -> w451
                    frame False {
                    }
                    frame True {
                    }
                  }
                  n298 = property on="TriggerSoftware" class="Bool"("DisabledEnum"=w451) -> ()  [unwired: 2 in, 2 out]
                }
                frame "曝光时间" {
                  n299 = local read "Open Status"() -> (w463:bool)
                  n300 = case shown="False" w463 {
                    tunnel: [T3."Disabled and Grayed Out" ("禁用") T3."Enabled" ("禁用")] -> w462
                    frame False {
                    }
                    frame True {
                    }
                  }
                  n301 = property on="ExposureTime" class="DigNum (strict)"("DisabledEnum"=w462) -> ()  [unwired: 2 in, 2 out]
                }
                frame "增益" {
                  n302 = local read "Open Status"() -> (w467:bool)
                  n303 = case shown="True" w467 {
                    tunnel: [T3."Disabled and Grayed Out" ("禁用") T3."Enabled" ("禁用")] -> w466
                    frame False {
                    }
                    frame True {
                    }
                  }
                  n304 = property on="Gain" class="DigNum (strict)"("DisabledEnum"=w466) -> ()  [unwired: 2 in, 2 out]
                }
                frame "自动白平衡" {
                  n305 = local read "Open Status"() -> (w472:bool)
                  n306 = local read "IsColor"() -> (w473:bool)
                  n307 = And(x=w472, y=w473) -> (x .and. y?=w471:bool)
                  n308 = case shown="True" w471 {
                    tunnel: [T3."Disabled and Grayed Out" ("禁用") T3."Enabled" ("禁用")] -> w470
                    frame False {
                    }
                    frame True {
                    }
                  }
                  n309 = property on="BalanceWhiteAuto" class="CmbBox"("DisabledEnum"=w470) -> ()  [unwired: 2 in, 2 out]
                }
              }
            }
            n310 = local read "IGxFactory"() -> (w412:refnum<k24>)
            n311 = call "UnInit.vi"("IGxFactory"=w412) -> ("error out"=w413:errorcluster)  [unwired: 1 in]
            n312 = Close Reference(reference=w412, error in (no error)=w413) -> ()  [unwired: 1 out]
          }
          frame "UpdateParam" {
            n313 = local read "Open Status"() -> (w486:bool)
            n314 = local read "IGxDevice"() -> (w482:refnum<k24>)
            n315 = Not A Number/Path/Refnum?(number/path/refnum=w482) -> (NaN/Path/Refnum?=w483:bool)
            n316 = Not(x=w483) -> (.not. x?=w485:bool)
            n317 = And(x=w485, y=w486) -> (x .and. y?=w484:bool)
            n318 = case shown="True" w484 {
              tunnel: [errorcluster {FALSE, 0, ""} w488] -> w479
              tunnel: string[] ["TriggerMode", "TriggerSource", "ExposureTime", "Gain", "BalanceWhiteAuto"] -> [_ w491]
              tunnel: w482 -> [_ w490]
              frame False {
              }
              frame True {
                n319 = for {
                  tunnel: w491 -> [w494] mode=indexing
                  tunnel: w490 -> [w493]
                  tunnel: [w492] -> w489 mode=indexing
                  n320 = case shown="\"BalanceWhiteAuto\"" w494 {
                    selector: w494 -> [w497 w501 w505 w509 w512]
                    tunnel: w493 -> [w498 w502 w506 w510 w513]
                    tunnel: [w495 w499 w503 w507 w515] -> w492
                    frame "TriggerMode", Default {
                      n321 = call "GetEnumValue.vi"("Feature Name"=w497, "IGxDevice"=w498) -> ("error out"=w495:errorcluster, "Enum Value"=w496:string)  [unwired: 1 in]
                      n322 = local write "TriggerMode"(w496) -> ()
                    }
                    frame "TriggerSource" {
                      n323 = call "GetEnumValue.vi"("Feature Name"=w501, "IGxDevice"=w502) -> ("error out"=w499:errorcluster, "Enum Value"=w500:string)  [unwired: 1 in]
                      n324 = local write "TriggerSource"(w500) -> ()
                    }
                    frame "ExposureTime" {
                      n325 = call "GetFloatValue.vi"("Feature Name"=w505, "IGxDevice"=w506) -> ("error out"=w503:errorcluster, "Float Value"=w504:dbl)  [unwired: 1 in]
                      n326 = local write "ExposureTime"(w504) -> ()
                    }
                    frame "Gain" {
                      n327 = call "GetFloatValue.vi"("Feature Name"=w509, "IGxDevice"=w510) -> ("error out"=w507:errorcluster, "Float Value"=w508:dbl)  [unwired: 1 in]
                      n328 = local write "Gain"(w508) -> ()
                    }
                    frame "BalanceWhiteAuto" {
                      n329 = call "IsImplemented.vi"("Feature Name"=w512, "IGxDevice"=w513) -> ("error out"=w514:errorcluster, "IsImplement"=w511:bool)  [unwired: 1 in]
                      n330 = case shown="True" w511 {
                        tunnel: [w516 w520] -> w515
                        tunnel: w514 -> [w516 w521]
                        tunnel: w513 -> [_ w518]
                        tunnel: w512 -> [_ w517]
                        frame False {
                        }
                        frame True {
                          n331 = call "GetEnumValue.vi"("error in (no error)"=w521, "Feature Name"=w517, "IGxDevice"=w518) -> ("error out"=w520:errorcluster, "Enum Value"=w519:string)
                          n332 = local write "BalanceWhiteAuto"(w519) -> ()
                        }
                      }
                      n333 = local write "IsColor"(w511) -> ()
                    }
                  }
                }
                n334 = Merge Errors(w489) -> (w488:errorcluster)
              }
            }
            n335 = Generate User Event(user event=w480, event data cluster="UpdateUI", error in=w479) -> (error out=w478:errorcluster)  [unwired: 1 in, 1 out]
            n336 = local write "error out"(w478) -> ()
            n337 = call <vilib>:"Simple Error Handler.vi"("error in (no error)"=w478) -> ()  [unwired: 4 in, 5 out]
          }
          frame "PicShow" {
            n338 = local read "Open Status"() -> (w528:bool)
            n339 = local read "IGxDevice"() -> (w524:refnum<k24>)
            n340 = Not A Number/Path/Refnum?(number/path/refnum=w524) -> (NaN/Path/Refnum?=w525:bool)
            n341 = Not(x=w525) -> (.not. x?=w527:bool)
            n342 = And(x=w527, y=w528) -> (x .and. y?=w526:bool)
            n343 = case shown="True" w526 {
              tunnel: [errorcluster {FALSE, 0, ""} errorcluster {FALSE, 0, ""}] -> w522
              tunnel: w524 -> [_ w534]
              frame False {
              }
              frame True {
                n344 = call "IsImplemented.vi"("Feature Name"="PixelColorFilter", "IGxDevice"=w534) -> ("IsImplement"=w536:bool)  [unwired: 1 in, 1 out]
                n345 = case shown="True" w536 {
                  tunnel: w534 -> [_ w543]
                  tunnel: [w537 w538] -> w531
                  frame False {
                    w537 = T4 0 items=["Grayscale (U8)", "Grayscale (I16)", "Grayscale (SGL)", "Complex (CSG)", "RGB (U32)", "HSL (U32)", "RGB (U64)", "Grayscale (U16)"] ("Image Type")
                  }
                  frame True {
                    n346 = call "GetEnumValue.vi"("Feature Name"="PixelColorFilter", "IGxDevice"=w543) -> ("Enum Value"=w541:string)  [unwired: 1 in, 1 out]
                    n347 = Equal?(x=w541, y="None") -> (x = y?=w539:bool)
                    n348 = case shown="False" w539 {
                      tunnel: [w544 w545] -> w538
                      frame False {
                        w544 = T4 4 items=["Grayscale (U8)", "Grayscale (I16)", "Grayscale (SGL)", "Complex (CSG)", "RGB (U32)", "HSL (U32)", "RGB (U64)", "Grayscale (U16)"] ("Image Type")
                      }
                      frame True {
                        w545 = T4 0 items=["Grayscale (U8)", "Grayscale (I16)", "Grayscale (SGL)", "Complex (CSG)", "RGB (U32)", "HSL (U32)", "RGB (U64)", "Grayscale (U16)"] ("Image Type")
                      }
                    }
                  }
                }
                n349 = call "IMAQ Create"("Image Name"="", "Image Type"=w531) -> ("New Image"=w532:T1)  [unwired: 3 in, 1 out]
                n350 = local write "Image Src"(w532) -> ()
              }
            }
            n351 = local write "error out"(w522) -> ()
            n352 = call <vilib>:"Simple Error Handler.vi"("error in (no error)"=w522) -> ()  [unwired: 4 in, 5 out]
          }
        }
      }
    }
  }
  n353 = while {
    tunnel: w2 -> [w551]
    tunnel: w1 -> [w546]
    stop <- w552 stop-if-true
    # "Acquisition Callback Function"
    n354 = Flush Event Queue(0:w551, 5:1) -> (8:w550:refnum<event-registration>, 11:w547:errorcluster)  [unwired: 4 in, 1 out]
    n355 = event shown="[1] <IFrameData>: User Event" {
      selector: w550 -> [_ _]
      dyn-events: _ -> [_ _]
      timeout: _ -> [_ _]
      tunnel: [_ FALSE] -> w552
      tunnel: [w553 w554] -> w548
      tunnel: w547 -> [w553 w557]
      tunnel: w546 -> [_ w560]
      event Timeout {
        n356 = event-data() -> ()  [unwired: 1 in, 3 out]
      }
      event User Event {
        n357 = event-data() -> ("IFrameData"=w562:refnum<k24>)  [unwired: 1 in, 4 out]
        n358 = flat-sequence {
          tunnel: w562 -> [w568]
          tunnel: [w568] -> w561
          tunnel: w560 -> [w567]
          tunnel: [w566] -> w558
          tunnel: w557 -> [w565]
          tunnel: [w564] -> w556
          tunnel: w561 -> [w573]
          tunnel: [w572] -> w559
          tunnel: w558 -> [w572]
          tunnel: w556 -> [w571]
          tunnel: [w570] -> w555
          tunnel: w559 -> [w607]
          tunnel: w555 -> [w606]
          tunnel: [w605] -> w554
          frame #0 {
            n359 = call <vilib>:"Acquire Semaphore.vi"("error in (no error)"=w565, "semaphore"=w567) -> ("error out"=w564:errorcluster, "semaphore out"=w566:T2)  [unwired: 3 in, 1 out]
          }
          frame #1 {
            n360 = local read "Acquisition Status"() -> (w569:bool)
            n361 = case shown="True" w569 {
              tunnel: [w574 w577] -> w570
              tunnel: w573 -> [_ w576]
              tunnel: w571 -> [w574 w575]
              frame False {
              }
              frame True {
                n362 = invoke class="IBaseData" method="GetStatus"(reference=w576, error in=w575) -> (reference out=w579:refnum<k24>, error out=w578:errorcluster, "GetStatus"=w580:i32)  [unwired: 1 in]
                n363 = case shown="0" w580 {
                  tunnel: [w581 w586] -> w577
                  tunnel: w579 -> [_ w582]
                  tunnel: w578 -> [w581 w583]
                  frame Default {
                  }
                  frame 0 {
                    n364 = local read "Image Src"() -> (w587:T1)
                    n365 = local read "Image Path"() -> (w585:path)
                    n366 = local read "ImageSaving"() -> (w590:bool)
                    n367 = call "GrabImageDisplay.vi"("error in (no error)"=w583, "Image Src"=w587, "IBaseData"=w582) -> ("error out"=w592:errorcluster, "Image out"=w584:T1)
                    "Image" <- w584
                    n368 = Not A Number/Path/Refnum?(number/path/refnum=w585) -> (NaN/Path/Refnum?=w588:bool)
                    n369 = Not(x=w588) -> (.not. x?=w589:bool)
                    n370 = And(x=w590, y=w589) -> (x .and. y?=w591:bool)
                    n371 = case shown="True" w591 {
                      tunnel: w585 -> [_ w600]
                      tunnel: w584 -> [_ w599]
                      tunnel: w592 -> [w593 w597]
                      tunnel: [w593 w596] -> w586
                      frame False {
                      }
                      frame True {
                        n372 = Path To String(path=w600) -> (string=w601:string)
                        n373 = Get Date/Time In Seconds() -> (seconds since 1Jan1904=w603:timestamp)
                        n374 = Concatenate Strings(w601, "\\%Y-%m-%d_%H_%M_%S%3u", ".jpg") -> (w602:string)
                        n375 = Format Date/Time String(time format string (%c)=w602, seconds (now)=w603) -> (date/time string=w604:string)  [unwired: 1 in]
                        n376 = String To Path(string=w604) -> (path=w598:path)
                        n377 = call "SaveImage.vi"("error in (no error)"=w597, "Path"=w598, "Image Src"=w599) -> ("error out"=w596:errorcluster)
                      }
                    }
                  }
                }
              }
            }
          }
          frame #2 {
            n378 = call <vilib>:"Release Semaphore.vi"("error in (no error)"=w606, "semaphore"=w607) -> ("error out"=w605:errorcluster)  [unwired: 4 in, 1 out]
          }
        }
      }
    }
    n379 = local write "error out"(w548) -> ()
  }
  n380 = Stop(stop? (T)=w4) -> ()
